vi "exercice5-2.vi"() -> ()   [LabVIEW 2013]
panel:
  out "Graphe":cluster{dbl, i32, dbl[]}(graph)
  # "Marche"
  # "Arret"
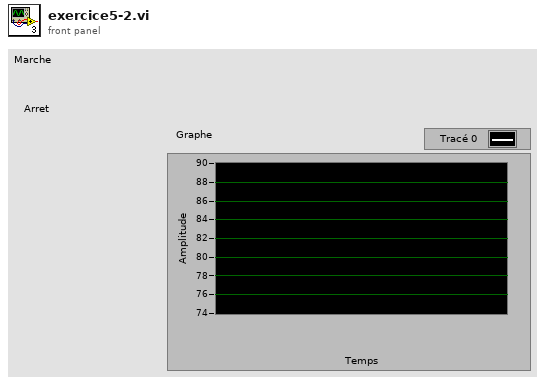
[diagram p1: front panel]
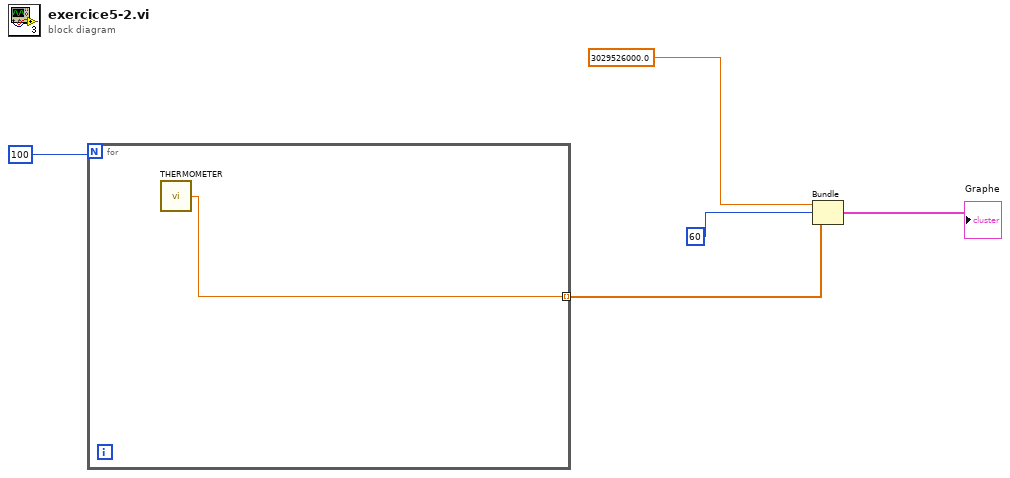
[diagram p0: block diagram]
diagram:
  n1 = for {
    N: 100 -> [_]
    tunnel: [w6] -> w2 mode=indexing
    n2 = call "THERMOMETER.vi"() -> ("temeperature"=w6:dbl)  [unwired: 1 in]
  }
  n3 = Bundle(3029526000.0, 60, w2) -> (→"Graphe":cluster{dbl, i32, dbl[]})  [unwired: 1 in]
